vi "Cluster Ref.vi"(8 "error in":errorcluster, 9 "Label Text":string, 10 "Input Array":string[](array[string]), 11 "Cluster Reference":refnum<vi>) -> (0 "error out":errorcluster, 2 "Array Out":string[](array[string]))   [LabVIEW 2022 SP3]
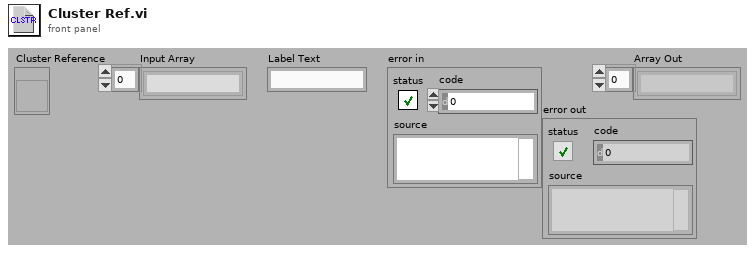
[diagram p1: front panel]
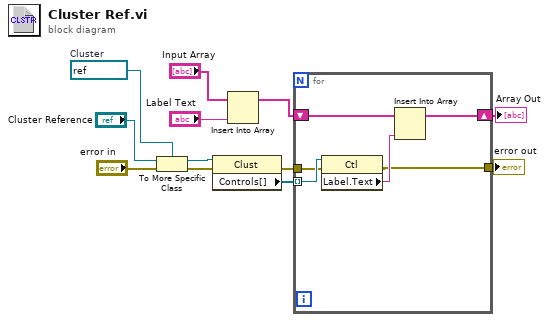
[diagram p0: block diagram]
diagram:
  w6 = refnum<vi> refnum  # Cluster
  n1 = To More Specific Class(target class=w6, reference="Cluster Reference", error in="error in") -> (specific class reference=w4:refnum<vi>, error out=w2:errorcluster)
  n2 = property class="Clust"(reference=w4, error in=w2) -> (error out=w11:errorcluster, "Controls[]"=w7:refnum<vi>[])  [unwired: 1 out]
  n3 = Insert Into Array(array="Input Array", new element="Label Text") -> (w9:string[])  [unwired: 1 in]
  n4 = for {
    tunnel: w7 -> [w18] mode=indexing
    shift-right: [w14] -> w10
    shift-left: w9 -> [w17]
    tunnel: w11 -> [w16]
    tunnel: [w13] -> w1
    n5 = property class="Ctl"(reference=w18, error in=w16) -> (error out=w13:errorcluster, "Label.Text"=w15:string)  [unwired: 1 out]
    n6 = Insert Into Array(array=w17, new element=w15) -> (w14:string[])  [unwired: 1 in]
  }
  "Array Out" <- w10
  "error out" <- w1
